vi "CRYZero pad trim off of array.vi"(11 "Array in":dbl[](array[numeric]) format="%.2f") -> (3 "Array out":dbl[](array[numeric]) format="%.2f")   [LabVIEW 2013]
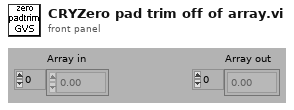
[diagram p1: front panel]
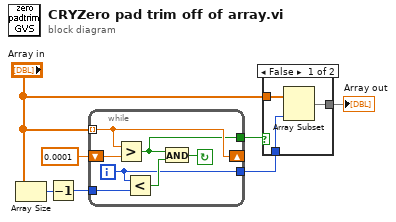
[diagram p0: block diagram]
diagram:
  n1 = Array Size(array="Array in") -> (size(s)=w7:i32)
  n2 = Decrement(x=w7) -> (x-1=w6:i32)
  n3 = while {
    tunnel: [w8] -> w1
    tunnel: [w9] -> w3
    shift-left: 0.0001 -> [w14]
    shift-right: [w13] -> _
    tunnel: w6 -> [w12]
    tunnel: "Array in" -> [w13] mode=indexing
    i -> [w9]
    stop <- w10 continue-if-true
    n4 = Greater?(x=w13, y=w14) -> (0:w8:bool)
    n5 = Less?(x=w9, y=w12) -> (x < y?=w11:bool)
    n6 = And(x=w8, y=w11) -> (x .and. y?=w10:bool)
  }
  n7 = case shown="False" w1 {
    tunnel: "Array in" -> [w17 w18]
    tunnel: w3 -> [w16 _]
    tunnel: [w15 w18] -> w2
    frame False {
      n8 = Array Subset(array=w17, length=w16) -> (w15:dbl[])  [unwired: 1 in]
    }
    frame True {
    }
  }
  "Array out" <- w2
